vi "File Extension and New Name.vi"(8 "error in":errorcluster, 9 "base template name":string, 10 "custom device name":string, 11 "filename":string) -> (0 "error out":errorcluster, 2 "extension":string, 3 "new filename":string)   [LabVIEW 2020, in "Template Tool.lvlib"]
uses:
  Template Tool.lvlib
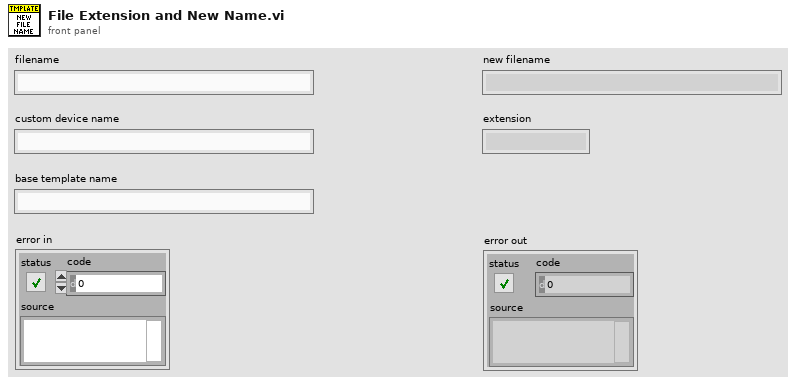
[diagram p1: front panel]
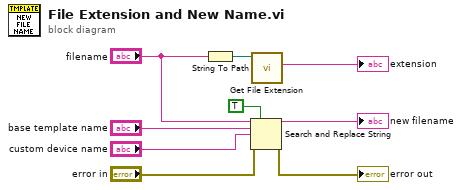
[diagram p0: block diagram]
diagram:
  n1 = String To Path(string="filename") -> (path=w4:path)
  n2 = Search and Replace String(replace all?=TRUE ("replace all? (F)"), input string="filename", search string="base template name", replace string="custom device name", error in="error in") -> (result string=→"new filename":string, error out=→"error out":errorcluster)  [unwired: 3 in, 2 out]
  n3 = call <vilib>:"Get File Extension.vi"("file"=w4) -> ("lowercase file extension"=→"extension":string)  [unwired: 6 in, 4 out]
